vi "Core Actor - Send Actor Message.vi"(8 "error in (no error)":errorcluster, 9 "Value":string, 11 "Parent_Class in":refnum<class "Message_Distributor_Class.lvclass">) -> (0 "error out":errorcluster, 3 "Parent_Class out":refnum<class "Message_Distributor_Class.lvclass">)   [LabVIEW 2023, in "Actor_Message_Distributor.lvlib" / "Message_Distributor_Class.lvclass"]
uses:
  Message_Distributor_Class.lvclass
  Distributor - Ctrl - Trigger Event Cluster.ctl
  Usr Ev/Distributor - Ctrl - Enum - Events.ctl
  Message_Distributor_Class.lvclass/Message_Distributor_Class.ctl
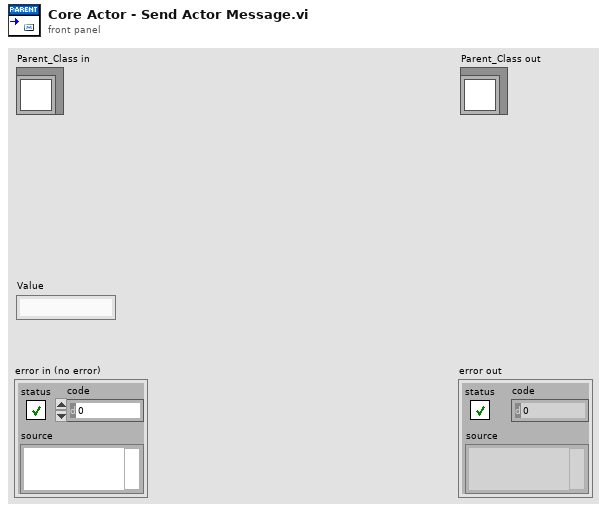
[diagram p1: front panel]
types:
  T1 = typedef "Actor_Message_Distributor.lvlib/Message_Distributor_Class.lvclass/Distributor - Ctrl - Trigger Event Cluster.ctl" = cluster{"Events":T2, "Data":string}
  T2 = typedef "Actor_Message_Distributor.lvlib/Message_Distributor_Class.lvclass/Distributor - Ctrl - Enum - Events.ctl" = enum16{"SEND MESSAGE Ev", "STOP_ACTOR Ev", "INIT_ACTOR Ev", "START Ev", "STOP Ev", "GET Ev", "SET Ev", "ERROR_HANDLER Ev", "RESET Ev", "DISPATCH MESSAGE 2 CHILDS Ev", "ECU RESET Ev"}
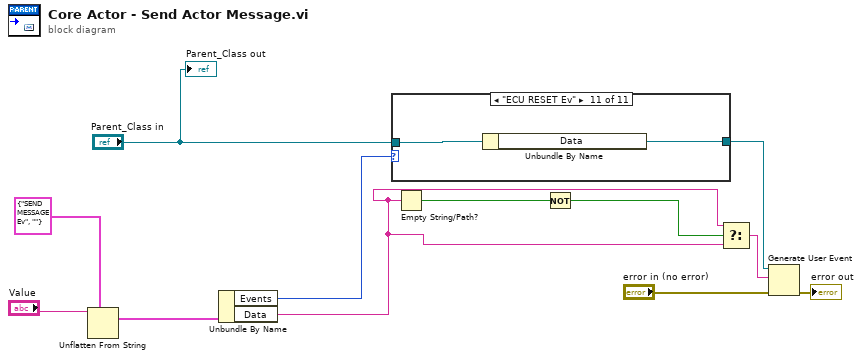
[diagram p0: block diagram]
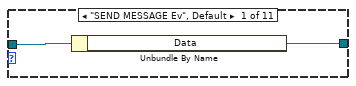
[diagram p2: hidden frame]
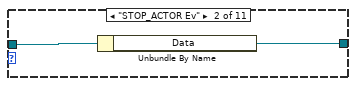
[diagram p3: hidden frame]
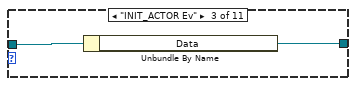
[diagram p4: hidden frame]
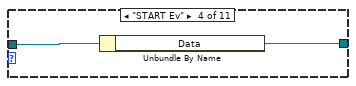
[diagram p5: hidden frame]
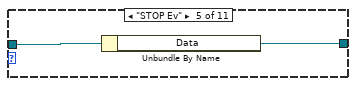
[diagram p6: hidden frame]
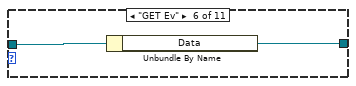
[diagram p7: hidden frame]
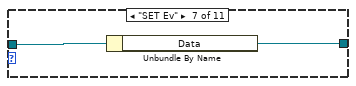
[diagram p8: hidden frame]
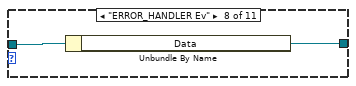
[diagram p9: hidden frame]
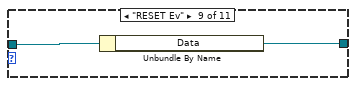
[diagram p10: hidden frame]
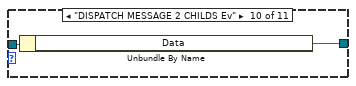
[diagram p11: hidden frame]
diagram:
  n1 = Unflatten From String(type=T1 {"Events"=enum."SEND MESSAGE Ev", "Data"=""} ("Cluster"), binary string="Value") -> (value=w5:T1)  [unwired: 3 in, 2 out]
  n2 = Unbundle By Name(w5) -> ("Events"=w4:T2, "Data"=w2:string)
  n3 = case shown="\"ECU RESET Ev\"" w4 {
    tunnel: "Parent_Class in" -> [w14 w16 w18 w20 w22 w24 w26 w28 w30 w32 w34]
    tunnel: [w13 w15 w17 w19 w21 w23 w25 w27 w29 w31 w33] -> w9
    frame "SEND MESSAGE Ev", Default {
      n4 = Unbundle By Name(w14) -> ("Data"=w13:refnum<user-event>)
    }
    frame "STOP_ACTOR Ev" {
      n5 = Unbundle By Name(w16) -> ("Data"=w15:refnum<user-event>)
    }
    frame "INIT_ACTOR Ev" {
      n6 = Unbundle By Name(w18) -> ("Data"=w17:refnum<user-event>)
    }
    frame "START Ev" {
      n7 = Unbundle By Name(w20) -> ("Data"=w19:refnum<user-event>)
    }
    frame "STOP Ev" {
      n8 = Unbundle By Name(w22) -> ("Data"=w21:refnum<user-event>)
    }
    frame "GET Ev" {
      n9 = Unbundle By Name(w24) -> ("Data"=w23:refnum<user-event>)
    }
    frame "SET Ev" {
      n10 = Unbundle By Name(w26) -> ("Data"=w25:refnum<user-event>)
    }
    frame "ERROR_HANDLER Ev" {
      n11 = Unbundle By Name(w28) -> ("Data"=w27:refnum<user-event>)
    }
    frame "RESET Ev" {
      n12 = Unbundle By Name(w30) -> ("Data"=w29:refnum<user-event>)
    }
    frame "DISPATCH MESSAGE 2 CHILDS Ev" {
      n13 = Unbundle By Name(w32) -> ("Data"=w31:refnum<user-event>)
    }
    frame "ECU RESET Ev" {
      n14 = Unbundle By Name(w34) -> ("Data"=w33:refnum<user-event>)
    }
  }
  n15 = Empty String/Path?(string/path=w2) -> (empty?=w12:bool)
  n16 = Not(x=w12) -> (.not. x?=w11:bool)
  n17 = Select(t=w2, s=w11, f=w2) -> (s? t:f=w8:string)
  n18 = Generate User Event(user event=w9, event data cluster=w8, error in="error in (no error)") -> (error out=→"error out":errorcluster)  [unwired: 1 in, 1 out]
  "Parent_Class out" <- "Parent_Class in"
